vi "Finalize.vi"(8 "error in":errorcluster, 11 "Plugin in":refnum<class "Configure Visa Device Channels.lvclass">) -> (0 "error out":errorcluster, 3 "Plugin out":refnum<class "Configure Visa Device Channels.lvclass">)   [LabVIEW 2026, in "Configure Visa Device Channels.lvlib" / "Configure Visa Device Channels.lvclass"]
uses:
  Configure Visa Device Channels.lvclass
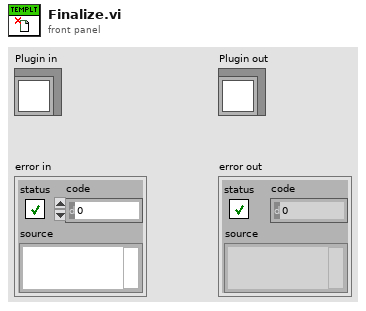
[diagram p1: front panel]
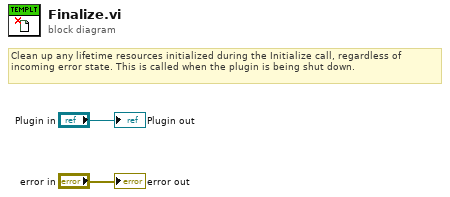
[diagram p0: block diagram]
diagram:
  # "Clean up any lifetime resources initialized during the Initialize call, regardless of incoming error state. This is called when the plugin is being shut down."
  "error out" <- "error in"
  "Plugin out" <- "Plugin in"
